vi "GetFrequencyTagId.vi"(8 "error in (no error)":errorcluster, 10 "tags":T1[](array[typedef]), 11 "VoltageBus  ChanID":string) -> (0 "error out":errorcluster, 3 "Frequency Tag ID":string)   [LabVIEW 2017, in "McsaUtilities.lvlib"]
uses:
  <vilib>/addons/InsightCM/Utilities/MCSA/McsaUtilities.lvlib
  <vilib>/addons/InsightCM/MessageBus/Base/controls/Tag.ctl
  <vilib>/addons/InsightCM/MessageBus/Base/controls/KeyValuePair.ctl
  <vilib>/addons/InsightCM/Utilities/PropertyHelpers/PropertyHelpers.lvlib
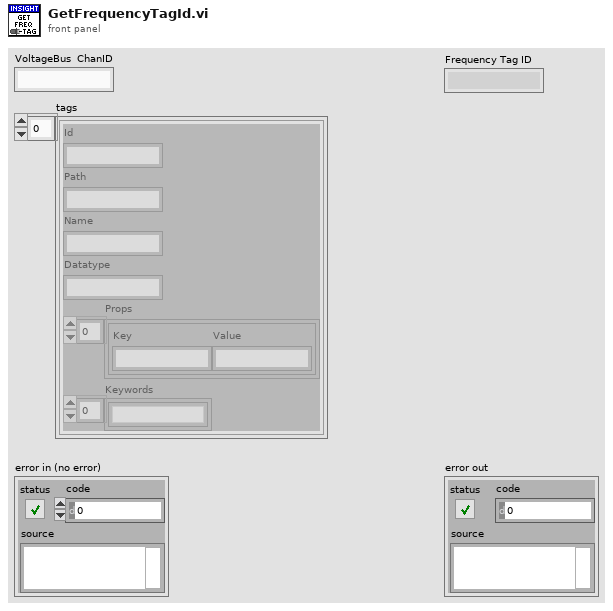
[diagram p1: front panel]
types:
  T1 = typedef "Tag.ctl" = cluster{"Id":string, "Path":string, "Name":string, "Datatype":string, "Props":T2[], "Keywords":string[]}
  T2 = typedef "KeyValuePair.ctl" = cluster{"Key":string, "Value":string}
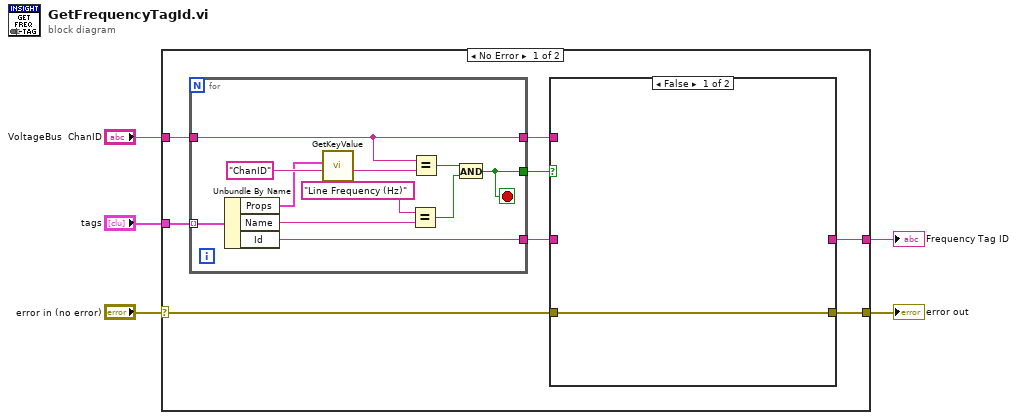
[diagram p0: block diagram]
diagram:
  n1 = case shown="No Error" "error in (no error)" {
    selector: "error in (no error)" -> [w9 w28]
    tunnel: "VoltageBus  ChanID" -> [w13 _]
    tunnel: "tags" -> [w12 _]
    tunnel: [w11 _] -> w1
    tunnel: [w10 w28] -> w2
    frame No Error {
      n2 = for {
        tunnel: w13 -> [w26]
        tunnel: w12 -> [w27] mode=indexing
        tunnel: [w26] -> w8
        tunnel: [w18] -> w7
        tunnel: [w17] -> w6
        stop <- w18 stop-if-true
        n3 = Unbundle By Name(w27) -> ("Props"=w23:T2[], "Name"=w21:string, "Id"=w17:string)
        n4 = call <vilib>:"GetKeyValue.vi"("key"="ChanID", "key value pairs"=w23) -> ("value"=w25:string)  [unwired: 7 in, 2 out]
        n5 = Equal?(x="Line Frequency (Hz)" ("key"), y=w21) -> (x = y?=w19:bool)
        n6 = Equal?(x=w26, y=w25) -> (x = y?=w20:bool)
        n7 = And(x=w20, y=w19) -> (x .and. y?=w18:bool)
      }
      n8 = case shown="False" w7 {
        tunnel: [_ w16] -> w11
        tunnel: w6 -> [_ w16]
        tunnel: [w14 w15] -> w10
        tunnel: w9 -> [w14 w15]
        tunnel: w8 -> [_ _]
        frame False {
        }
        frame True {
        }
      }
    }
    frame Error {
    }
  }
  "error out" <- w2
  "Frequency Tag ID" <- w1
